vi "do_Taring_Weighing_Machine.vi"(8 "error in (no error)":errorcluster, 11 "Waage_Config":T1={"Enable Termination\nChar (T)"=TRUE, "termination char\n(0xA = '\\n' = LF) "=10, "timeout (10sec)"=3000, "baud rate (9600)"=9600, "data bits (8)"=8, "parity (0:none)"=enum."None", "stop bits (10: 1 bit)"=10, "flow control (0:none)"=0, "Serial Port"=""} {"flow control (0:none)" items=["None", "XON/XOFF", "RTS/CTS", "XON/XOFF & RTS/CTS", "DTR/DSR", "XON/XOFF & DTR/DSR"]; "stop bits (10: 1 bit)" items=["1.0"=10, "1.5"=15, "2.0"=20]}) -> (0 "error out":errorcluster)   [LabVIEW 2012]
uses:
  <vilib>/Instr/_visa.llb/VISA Configure Serial Port (Instr).vi
panel:
  out "return count 2":u32
  out "return count":u32
  out "read buffer":string
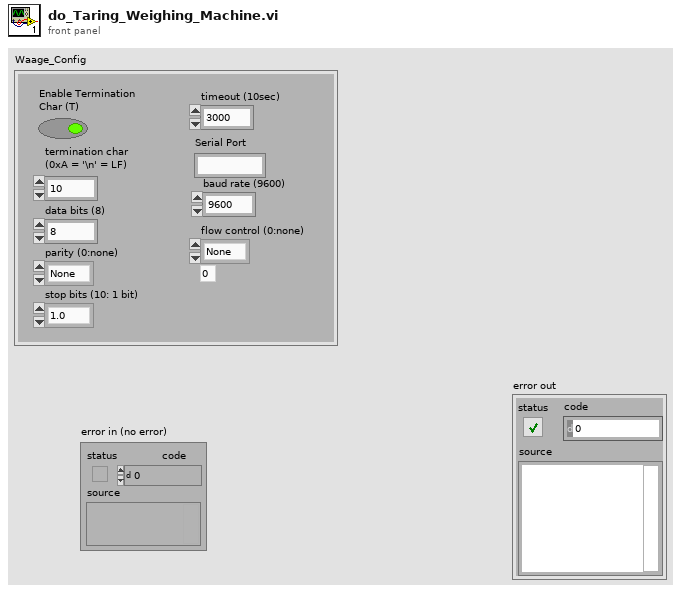
[diagram p1: front panel]
types:
  T1 = cluster{"Enable Termination\nChar (T)":bool, "termination char\n(0xA = '\\n' = LF) ":u8, "timeout (10sec)":u32, "baud rate (9600)":u32, "data bits (8)":u16, "parity (0:none)":enum16{"None", "Odd", "Even", "Mark", "Space"}, "stop bits (10: 1 bit)":u16, "flow control (0:none)":u16, "Serial Port":string}
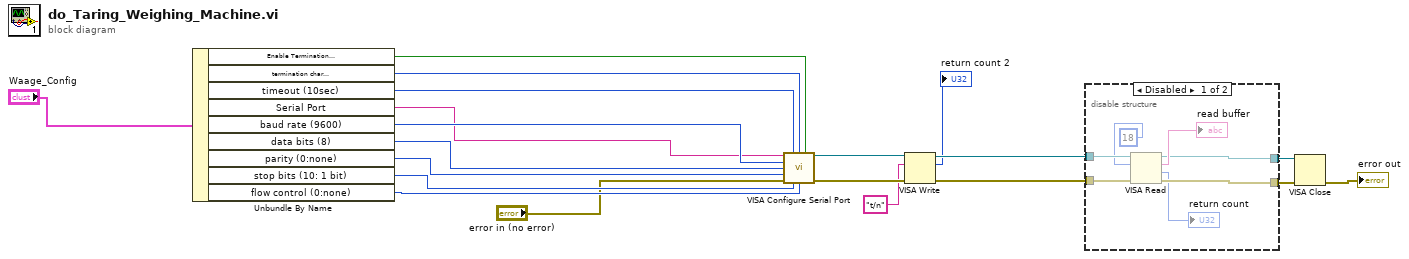
[diagram p0: block diagram]
diagram:
  n1 = Unbundle By Name("Waage_Config") -> ("Enable Termination\nChar (T)"=w12:bool, "termination char\n(0xA = '\\n' = LF)"=w11:u8, "timeout (10sec)"=w10:u32, "Serial Port"=w1:string, "baud rate (9600)"=w9:u32, "data bits (8)"=w8:u16, "parity (0:none)"=w7:enum16{"None", "Odd", "Even", "Mark", "Space"}, "stop bits (10: 1 bit)"=w6:u16, "flow control (0:none)"=w5:u16)
  n2 = call-poly "VISA Configure Serial Port"("VISA resource name"=w1, "timeout (10sec)"=w10, "termination char\n(0xA = '\\n' = LF)"=w11, "Enable Termination\nChar (T)"=w12, "baud rate (9600)"=w9, "data bits (8)"=w8, "parity (0:none)"=w7, "error in (no error)"="error in (no error)", "stop bits (10: 1 bit)"=w6, "flow control (0:none)"=w5) -> ("VISA resource name out"=w20:refnum<visa-resource-name>, "error out"=w19:errorcluster)  [unwired: 4 in]
  n3 = VISA Write(VISA resource name=w20, write buffer="t/n", error in (no error)=w19) -> (VISA resource name out=w18:refnum<visa-resource-name>, return count=→"return count 2":u32, error out=w17:errorcluster)
  n4 = disable-structure shown="Disabled" {
    disable-tunnel: w18 -> [w27 w29]
    disable-tunnel: w17 -> [w26 w28]
    disable-tunnel: [w24 w29] -> w16
    disable-tunnel: [w23 w28] -> w15
    frame Disabled {
      n5 = VISA Read(VISA resource name=w27, byte count=u32 18, error in (no error)=w26) -> (VISA resource name out=w24:refnum<visa-resource-name>, read buffer=→"read buffer":string, return count=→"return count":u32, error out=w23:errorcluster)
    }
    frame Enabled {
    }
  }
  n6 = VISA Close(VISA resource name=w16, error in (no error)=w15) -> (error out=→"error out":errorcluster)
